vi "Process.vi"(8 "error in":errorcluster, 11 "Measurement.Free.UI":refnum<class "Measurement.Free.UI.lvclass">) -> (0 "error out":errorcluster, 3 "Measurement.Free.UI out":refnum<class "Measurement.Free.UI.lvclass">)   [LabVIEW 2017, in "Measurement.Free.UI.lvclass"]
doc: "---------------------------------------------------------------\nJKI State Machine Objects™\nhttp://jki.net/state-machine-objects/\nCopyright (C) 2005-2015, JKI <info@jki.net>\nALL RIGHTS RESERVEDJKI State Machine Objects (SMO) 1.0.0.5\nJKI - JKI\nCopyright (c) 2016, JKI"
uses:
  Measurement.Free.UI.lvclass
  D:/Program Files (x86)/National Instruments/LabVIEW 2017/vi.lib/JKI/JKI SMO/SMO/SMO.lvclass
  D:/Program Files (x86)/National Instruments/LabVIEW 2017/vi.lib/JKI/JKI SMO/SMO.UI/SMO.UI.lvclass
  <vilib>/JKI/JKI SMO/SMO/Typedefs/Parent Call--Enum.ctl
  Measurement.Free/Measurement.Free.lvclass
  D:/upwork/Laser Measurement Tool/Laser/project/Subsystems/Measurement/Measurement.lvclass
  Measurement.UI/Measurement.UI.lvclass
  <vilib>/JKI/JKI SMO/SMO/SMO.lvclass
  <vilib>/JKI/JKI SMO/SMO.UI/SMO.UI.lvclass
  Measurement/Measurement.lvclass
panel:
  in  "Set OPA Wavelength":bool
  in  "Set SMU Votage":bool
  in  "Shutter":bool
  in  "Wavelength, nm:":dbl=620.0
  in  "SMU Voltage, V:":dbl=1.0
  out "Initialized":bool
  out "Power monitor":cluster{"X":dbl, "Y":dbl}[](graph) caption="XY Graph - Dark"
  out "SMU":cluster{"X":dbl, "Y":dbl}[](graph) caption="XY Graph - Dark"
  out "LIA":cluster{"X":dbl, "Y":dbl}[](graph) caption="XY Graph - Dark"
  in  "Clear Button":bool
  in  "Pause Button":bool
  in  "Stop Button":bool
  in  "Start Button":bool
  in  "Close Button":bool
  # "SMU Control"
  # "OPA Control"
  # "For instructions on how to use the JKI State Machine Objects, examples and video tutorials, visit:\nhttp://jki.net/state-machine-objects/\n\nJKI State Machine Objects™\nhttp://jki.net/state-machine-objects/\nCopyright (C) 2005-2015, JKI <info@jki.net>\nALL RIGHTS RESERVED"
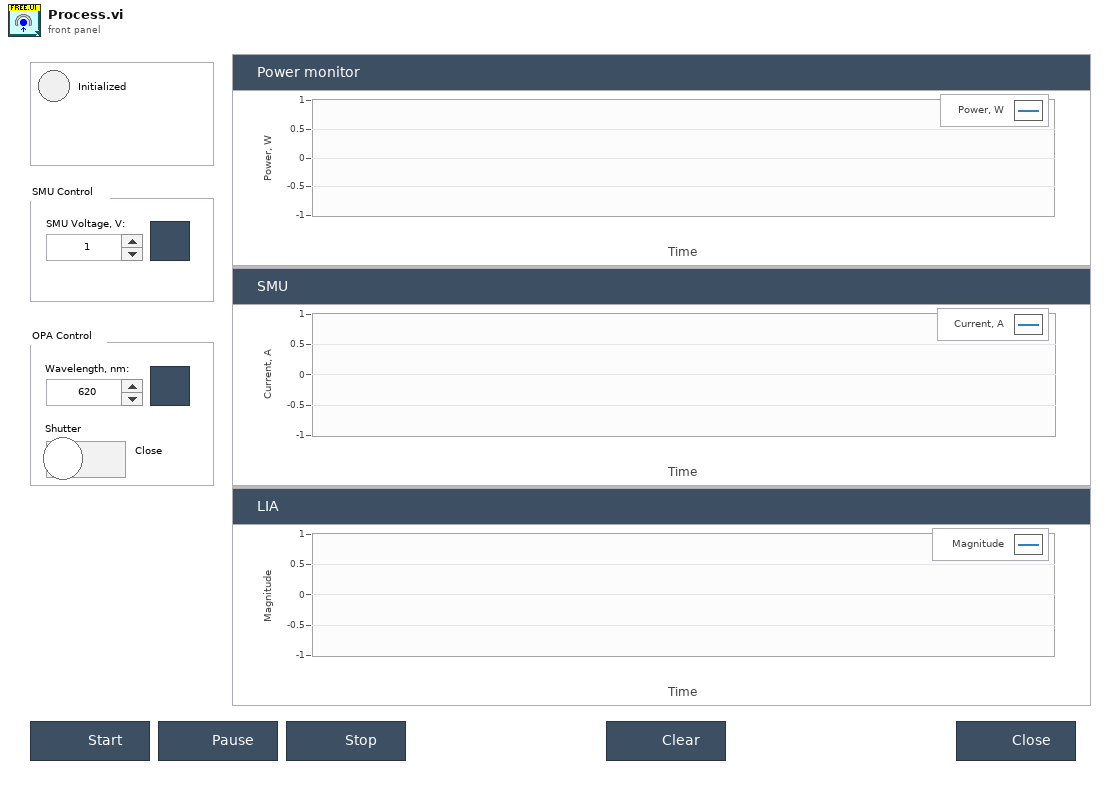
[diagram p1: front panel]
types:
  T1 = typedef "SMO.lvclass/Parent Call--Enum.ctl" = enum16{"Allows parent to run", "Does not request parent to run"}
  T2 = enum32{"invalid app kind", "Development System", "Run Time System", "Student Edition", "Embedded LabVIEW", "Evaluation", "Custom"}
  T3 = enum32{"Invalid", "Standard", "Closed", "Hidden", "Minimized", "Maximized"}
  T4 = typedef "Measurement.lvclass/PublicEvents--Measurement.Initialized.ctl" = bool
  T5 = enum8{"Enabled", "Disabled", "Disabled and Grayed Out"}
  T6 = typedef "Measurement.Free.UI.lvclass/Dependencies--Cluster.ctl" = cluster{"Measurement.Free":refnum<class "Measurement.Free.lvclass">}
  T7 = cluster{"Core":cluster{"Current VI Reference":refnum<vi>, "Close Panel on Exit?":bool, "error":errorcluster}, "Self Reference":refnum<class "Measurement.Free.UI.lvclass">, "Dependencies":T6, "SMU Data":cluster{"X":dbl, "Y":dbl}[], "LIA Data":cluster{"X":dbl, "Y":dbl}[], "OPM Data":cluster{"X":dbl, "Y":dbl}[]}
  T8 = cluster{"Current VI Reference":refnum<vi>, "Close Panel on Exit?":bool, "error":errorcluster}
  T9 = typedef "SMO.lvclass/Protected Events.ctl" = cluster{"StopProcesses":refnum<user-event>, "AbortProcesses":refnum<user-event>, "Config Changed":refnum<user-event>, "Dependency":refnum<user-event>}
  T10 = cluster{"Event Registration Refnum":refnum<event-registration>, "Measurement Public Events":refnum<event-registration>}
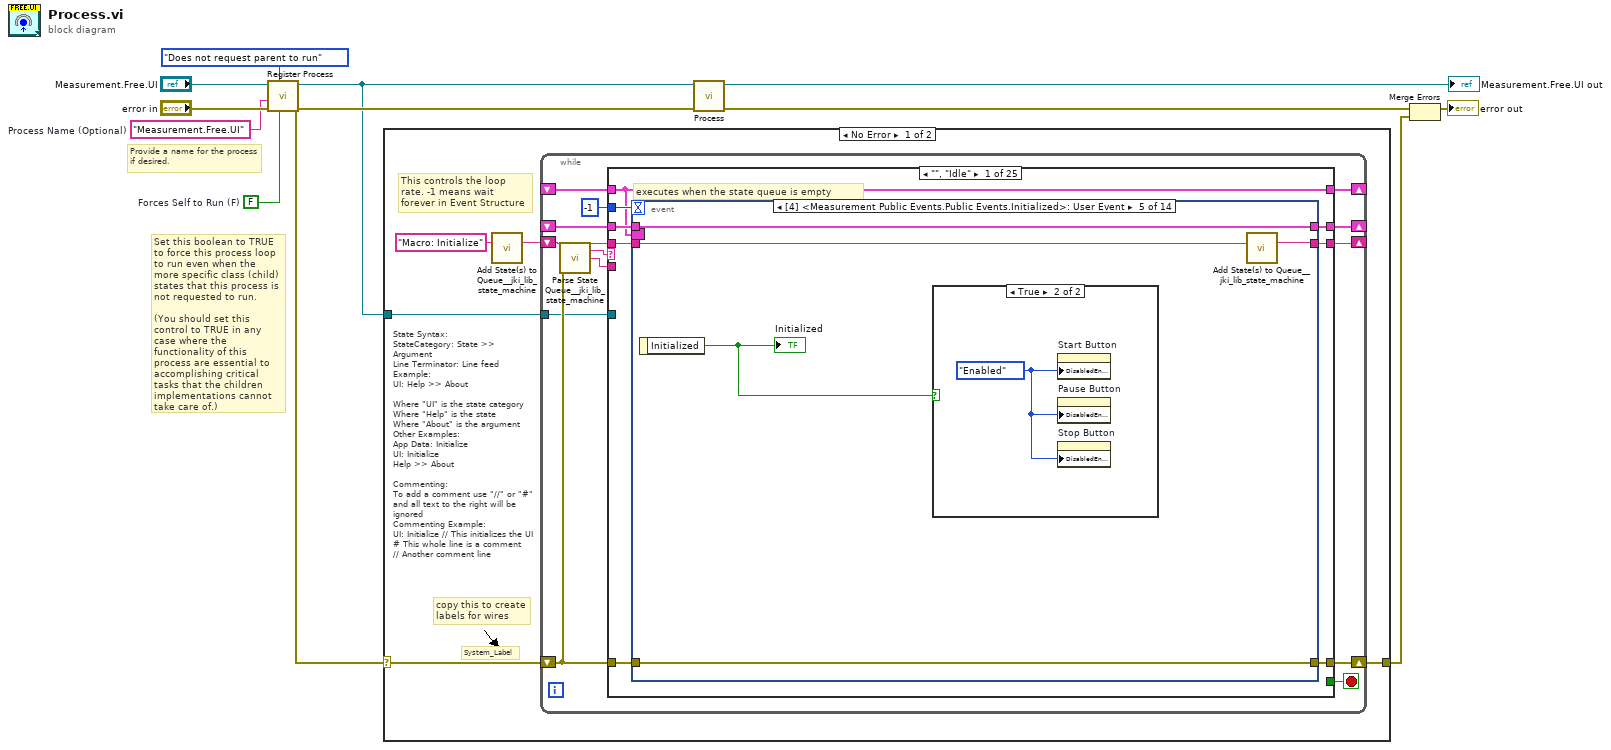
[diagram p0: block diagram]
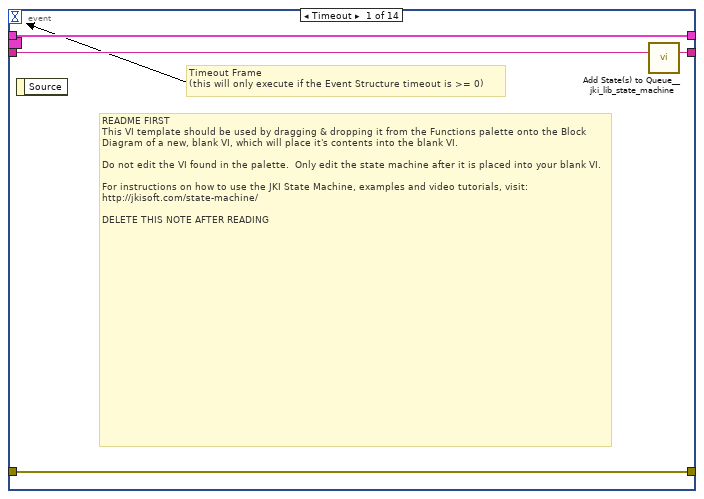
[diagram p2: hidden frame]
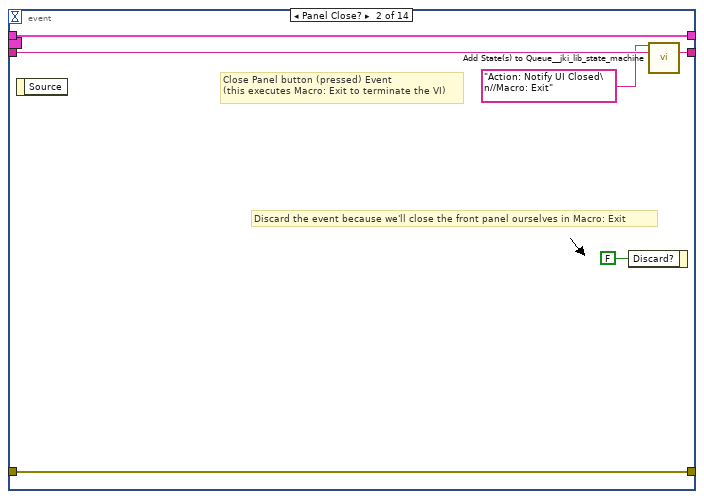
[diagram p3: hidden frame]
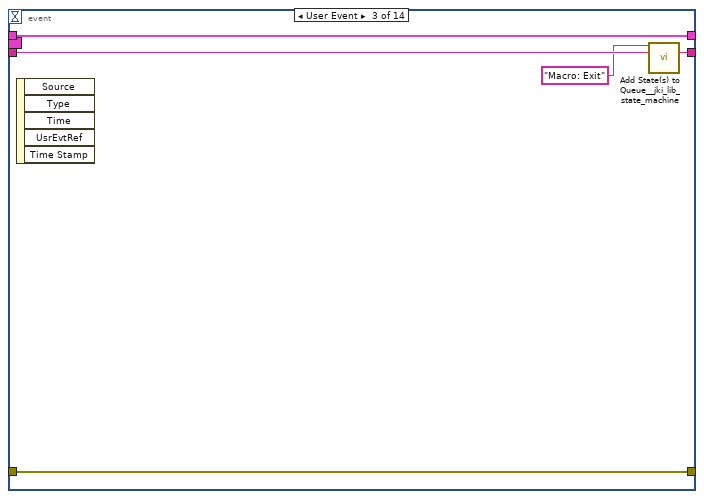
[diagram p4: hidden frame]
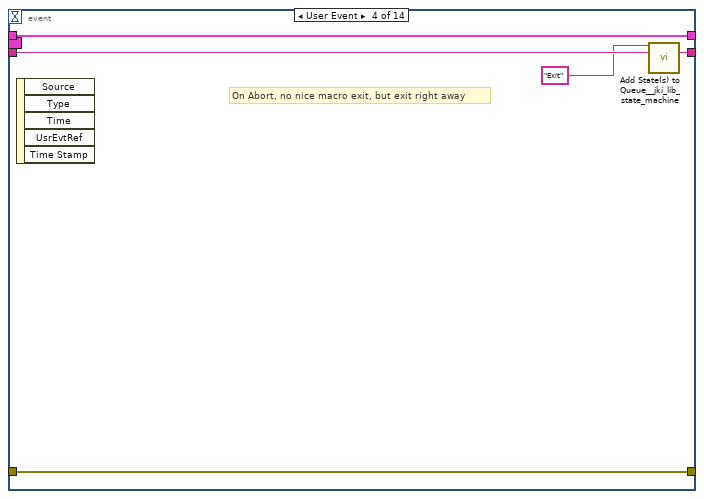
[diagram p5: hidden frame]
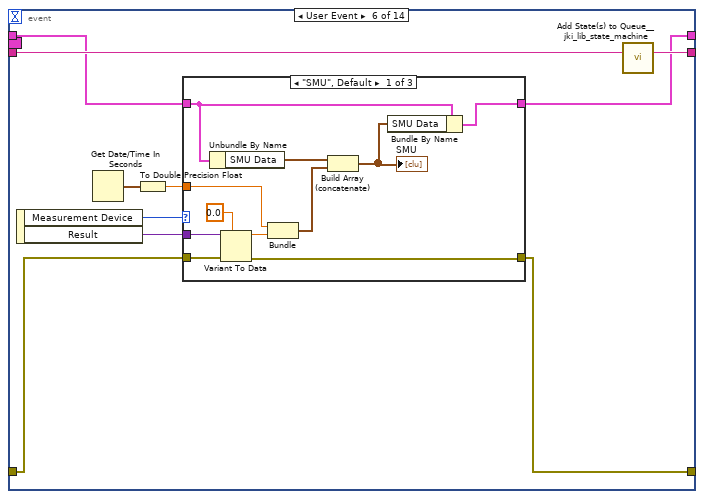
[diagram p7: hidden frame]
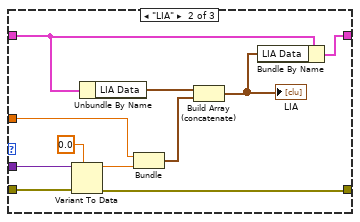
[diagram p8: hidden frame]
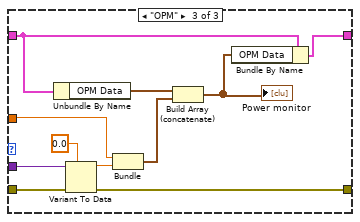
[diagram p9: hidden frame]
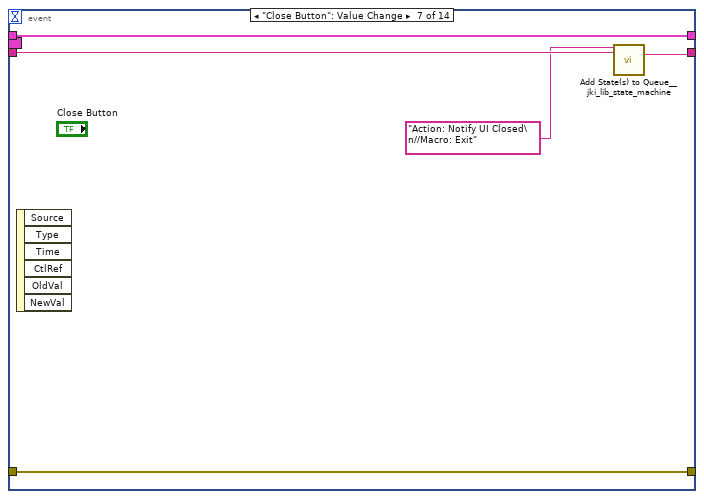
[diagram p10: hidden frame]
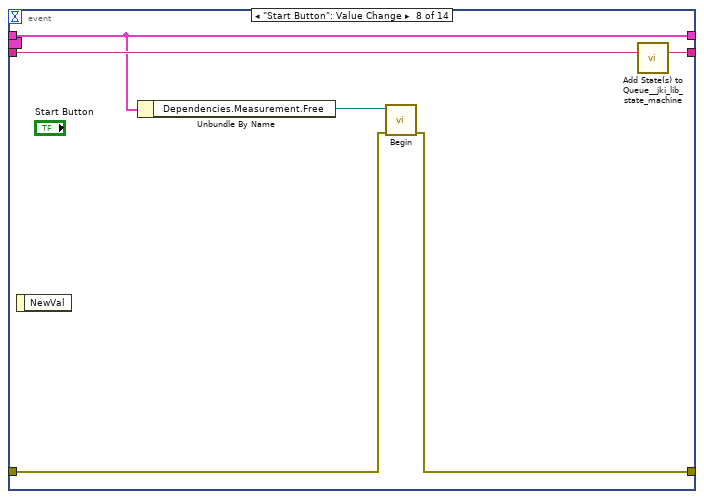
[diagram p11: hidden frame]
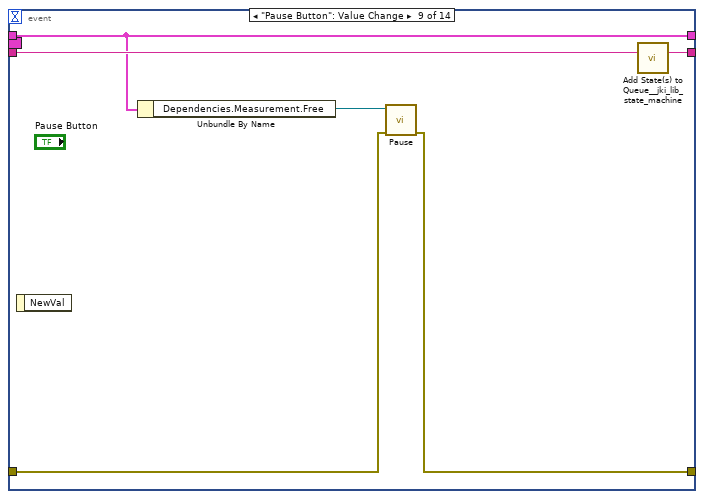
[diagram p12: hidden frame]
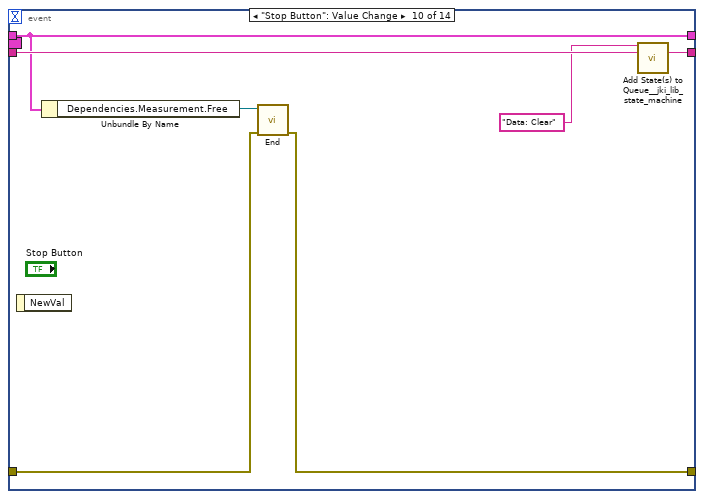
[diagram p13: hidden frame]
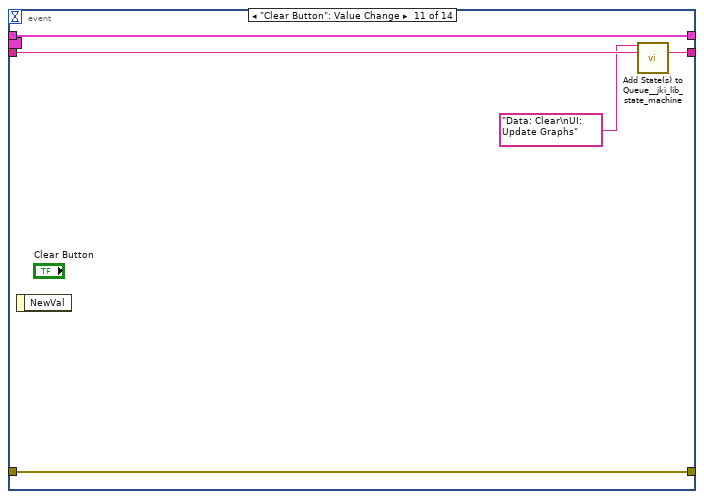
[diagram p14: hidden frame]
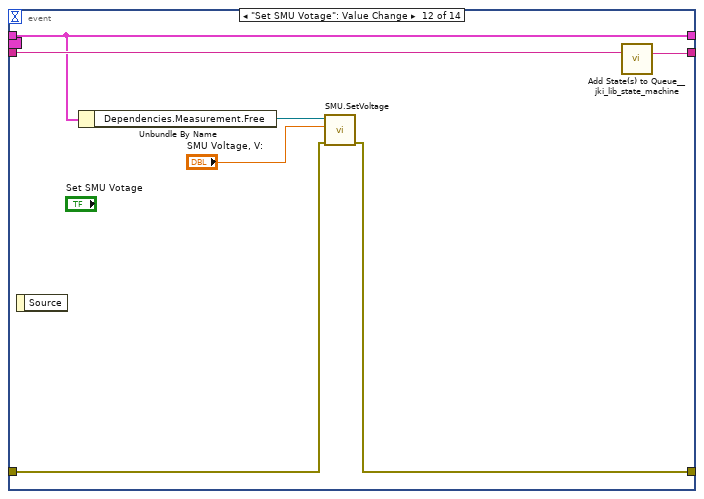
[diagram p15: hidden frame]
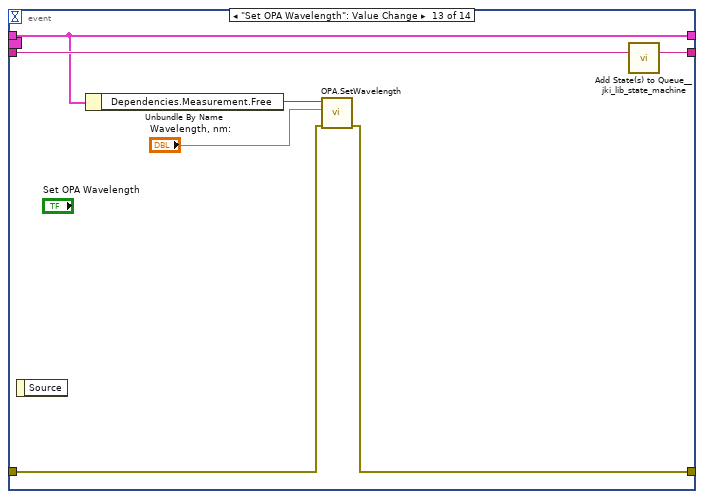
[diagram p16: hidden frame]
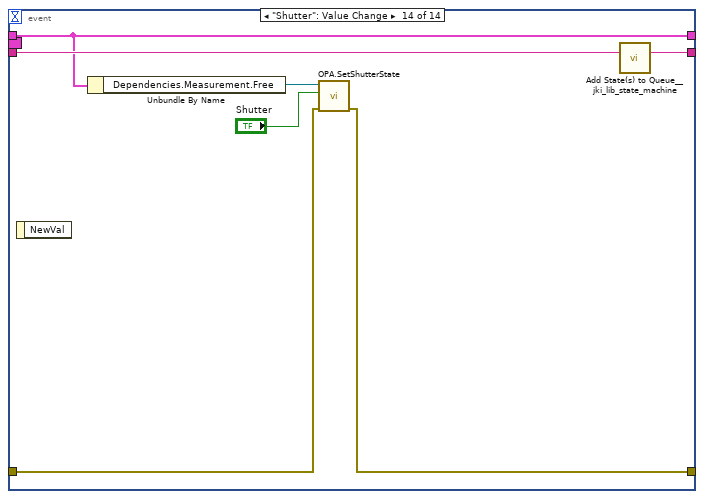
[diagram p17: hidden frame]
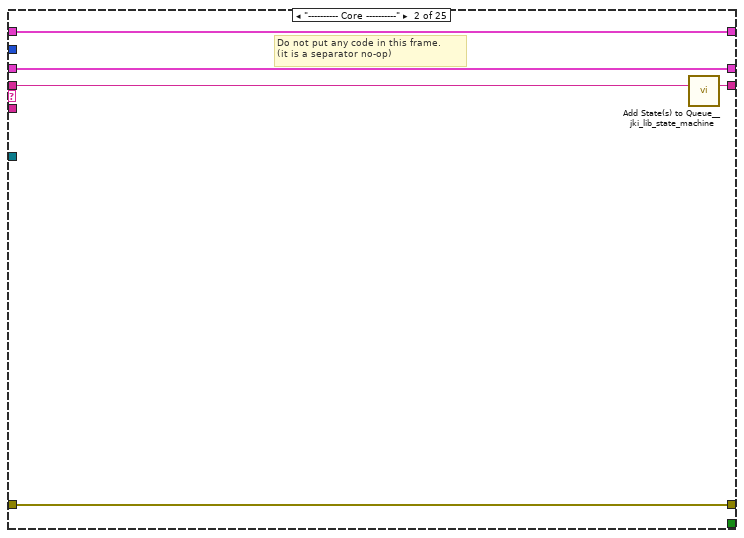
[diagram p18: hidden frame]
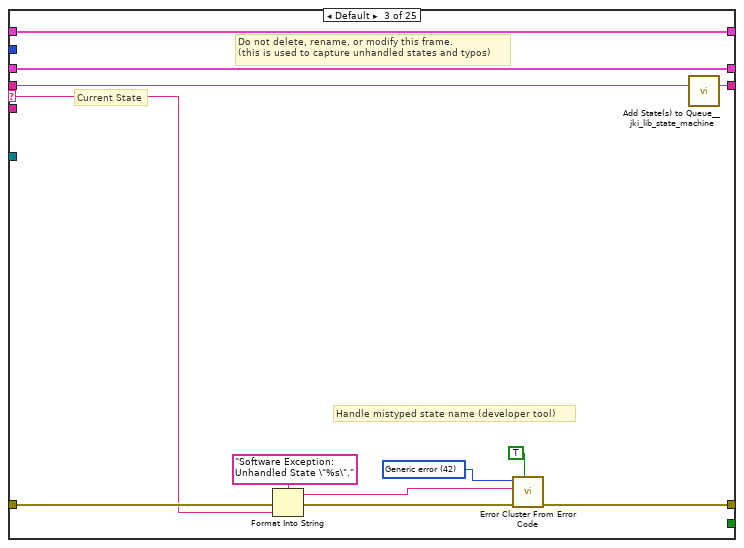
[diagram p19: hidden frame]
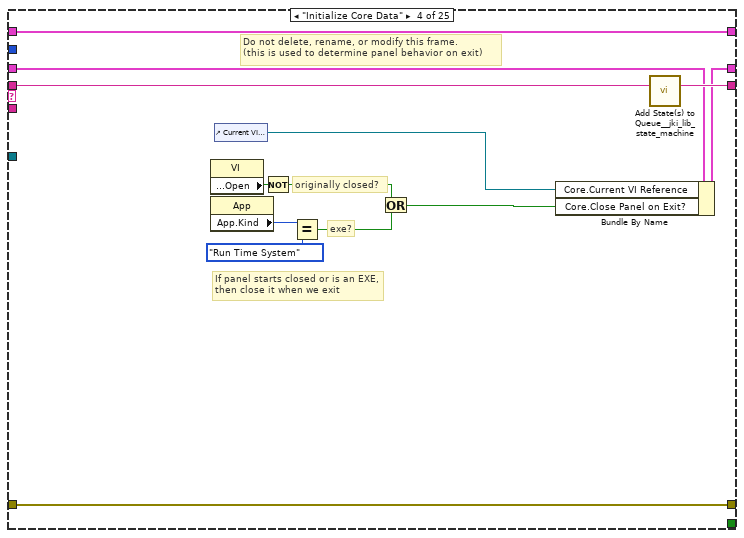
[diagram p20: hidden frame]
diagram:
  w2 = FALSE  # Forces Self to Run (F)
  w1 = "Measurement.Free.UI"  # Process Name (Optional)
  # "Provide a name for the process\nif desired."
  # "Set this boolean to TRUE to force this process loop to run even when the more specific class (child) states that this process is not requested to run.\n\n(You should set this control to TRUE in any case where the functionality of this process are essential to accomplishing critical tasks that the children implementations cannot take care of.)"
  n1 = call <vilib>:"Register Process.vi"("Forces Self to Run (F)"=w2, "Parent Call"=Parent_Call--Enum."Does not request parent to run", "error in (no error)"="error in", "Process Name (optional)"=w1, "SMO"="Measurement.Free.UI") -> ("error out"=w8:errorcluster, "SMO out"=w7:refnum<class "Measurement.Free.UI.lvclass">)  [unwired: 5 in]
  n2 = case shown="No Error" w8 {
    selector: w8 -> [w13 w402]
    tunnel: w7 -> [w14 _]
    tunnel: [w12 w402] -> w4
    frame No Error {
      # "State Syntax:\nStateCategory: State >> Argument\nLine Terminator: Line feed\nExample:\nUI: Help >> About\n\nWhere \"UI\" is the state category\nWhere \"Help\" is the state\nWhere \"About\" is the argument\nOther Examples:\nApp Data: Initialize\nUI: Initialize\nHelp >> About\n\nCommenting:\nTo add a comment use \"//\" or \"#\" and all text to the right will be ignored\nCommenting Example:\nUI: Initialize // This initializes the UI\n# This whole line is a comment\n// Another comment line"
      # "copy this to create labels for wires"
      # "This controls the loop rate. -1 means wait forever in Event Structure"
      # "System_Label"
      n3 = call <vilib>:"Add State(s) to Queue__jki_lib_state_machine.vi"("State(s) in (\"\")"="Macro: Initialize") -> ("States Out"=w16:string)  [unwired: 14 in]
      n4 = while {
        shift-right: [w23] -> _
        shift-left: _ -> [w22]
        shift-right: [w26] -> w12
        shift-left: w13 -> [w20]
        shift-right: [w25] -> _
        shift-left: w16 -> [w27]
        tunnel: w14 -> [w19]
        shift-right: [w18] -> _
        shift-left: _ -> [w17]
        stop <- w24 stop-if-true
        n5 = call <vilib>:"Parse State Queue__jki_lib_state_machine.vi"("State Queue"=w27, "Error In (no error)"=w20) -> ("Remaining States"=w29:string, "Current State"=w30:string, "Arguments"=w28:string)  [unwired: 11 in]
        n6 = case shown="\"\", \"Idle\"" w30 {
          selector: w30 -> [_ _ w164 _ _ _ _ _ _ _ _ _ _ _ _ _ _ _ _ _ _ _ _ _ _]
          tunnel: w29 -> [w38 w162 w168 w187 w201 w207 w212 w227 w234 w241 w246 w256 w263 w279 w318 w323 w332 w346 w351 w362 w367 w381 w387 w394 w401]
          tunnel: w28 -> [_ _ _ _ _ _ _ _ _ _ _ _ w257 w273 _ _ _ _ _ _ _ _ _ _ _]
          tunnel: w22 -> [w36 w159 w166 w178 w190 w203 w209 _ w230 w236 w243 w254 w261 w275 w315 w320 w328 w337 w348 w359 w364 w373 w385 w390 w397]
          tunnel: [w35 w160 w170 w184 w192 w202 w210 w217 w232 w237 w244 w250 w258 w276 w307 w321 w330 w344 w349 w353 w365 w376 w382 w391 w395] -> w26
          tunnel: w20 -> [w34 w160 w169 w184 w197 _ w210 w224 w232 w238 w244 w248 w259 w277 w311 w321 w330 w344 w349 w354 w365 w378 w383 w391 w396]
          tunnel: [w37 w161 w167 w186 w200 w206 w211 w226 w233 w240 w245 w255 w262 w278 w317 w322 w331 w345 w350 w361 w366 w380 w386 w393 w400] -> w25
          tunnel: [_ _ _ _ _ TRUE _ _ _ _ _ _ _ _ _ _ _ _ _ _ _ _ _ _ _] -> w24
          tunnel: [w33 w159 w166 w185 w189 w203 w209 w225 w228 w236 w243 w254 w261 w275 w315 w320 w328 w337 w348 w359 w364 w373 w385 w389 w397] -> w23
          tunnel: -1 ("Timeout") -> [w32 _ _ _ _ _ _ _ _ _ _ _ _ _ _ _ _ _ _ _ _ _ _ _ _]
          tunnel: w19 -> [_ _ _ _ _ _ _ w222 _ _ _ _ _ _ _ _ _ _ _ _ _ _ _ _ _]
          tunnel: [w31 w158 w163 w175 w199 w204 w208 w221 w231 w235 w242 w253 w260 w272 w316 w319 w329 w338 w347 w360 w363 w371 w384 w392 w399] -> w18
          tunnel: w17 -> [w31 w158 w163 w175 w199 w204 w208 w221 w231 w235 w242 w253 w260 w272 w316 w319 w329 w338 w347 w360 w363 _ w384 w392 w399]
          frame "", "Idle" {
            # "executes when the state queue is empty"
            n7 = event shown="[4] <Measurement Public Events.Public Events.Initialized>: User Event" {
              selector: w31 -> [_ _ _ _ _ _ _ _ _ _ _ _ _ _]
              dyn-events: _ -> [_ _ _ _ _ _ _ _ _ _ _ _ _ _]
              timeout: w32 -> [_ _ _ _ _ _ _ _ _ _ _ _ _ _]
              tunnel: w38 -> [w42 w48 w53 w58 w61 w73 w110 w118 w124 w131 w136 w142 w149 w156]
              tunnel: [w41 w47 w52 w57 w62 w74 w111 w117 w123 w130 w135 w143 w150 w157] -> w37
              tunnel: w36 -> [w39 w44 w50 w55 w63 w70 w109 w116 w122 w129 w134 w141 w148 w155]
              tunnel: [w40 w43 w51 w56 w60 w65 w112 w113 w119 w126 w132 w137 w144 w151] -> w35
              tunnel: w34 -> [w40 w43 w51 w56 w60 w66 w112 w114 w120 w127 w132 w138 w145 w152]
              tunnel: [w39 w44 w50 w55 w63 w69 w109 w116 w122 w129 w134 w141 w148 w155] -> w33
              event Timeout {
                # "README FIRST\nThis VI template should be used by dragging & dropping it from the Functions palette onto the Block Diagram of a new, blank VI, which will place it's contents into the blank VI.\n\nDo not edit the VI found in the palette.  Only edit the state machine after it is placed into your blank VI.\n\nFor instructions on how to use the JKI State Machine, examples and video tutorials, visit:\nhttp://jkisoft.com/state-machine/\n\nDELETE THIS NOTE AFTER READING"
                # "Timeout Frame\n(this will only execute if the Event Structure timeout is >= 0)"
                n8 = event-data() -> ()  [unwired: 1 in, 1 out]
                n9 = call <vilib>:"Add State(s) to Queue__jki_lib_state_machine.vi"("State(s) in (\"\")"=w42) -> ("States Out"=w41:string)  [unwired: 14 in]
              }
              event Panel Close? {
                # "Discard the event because we'll close the front panel ourselves in Macro: Exit"
                # "Close Panel button (pressed) Event\n(this executes Macro: Exit to terminate the VI)"
                n10 = event-data() -> ()  [unwired: 1 in, 1 out]
                n11 = event-data("Discard?"=FALSE) -> ()  [unwired: 1 in, 1 out]
                n12 = call <vilib>:"Add State(s) to Queue__jki_lib_state_machine.vi"("State(s) in Front (\"\")"="Action: Notify UI Closed\n//Macro: Exit", "State(s) in (\"\")"=w48) -> ("States Out"=w47:string)  [unwired: 13 in]
              }
              event User Event {
                n13 = event-data() -> ()  [unwired: 1 in, 5 out]
                n14 = call <vilib>:"Add State(s) to Queue__jki_lib_state_machine.vi"("State(s) in Front (\"\")"="Macro: Exit", "State(s) in (\"\")"=w53) -> ("States Out"=w52:string)  [unwired: 13 in]
              }
              event User Event {
                # "On Abort, no nice macro exit, but exit right away"
                n15 = event-data() -> ()  [unwired: 1 in, 5 out]
                n16 = call <vilib>:"Add State(s) to Queue__jki_lib_state_machine.vi"("State(s) in Front (\"\")"="Exit", "State(s) in (\"\")"=w58) -> ("States Out"=w57:string)  [unwired: 13 in]
              }
              event User Event {
                n17 = event-data() -> ("Initialized"=w59:T4)  [unwired: 1 in]
                "Initialized" <- w59
                n18 = case shown="True" w59 {
                  frame False {
                  }
                  frame True {
                    w64 = T5."Enabled" ("Disabled")
                    n19 = property on="Start Button" class="Bool"("DisabledEnum"=w64) -> ()  [unwired: 2 in, 2 out]
                    n20 = property on="Pause Button" class="Bool"("DisabledEnum"=w64) -> ()  [unwired: 2 in, 2 out]
                    n21 = property on="Stop Button" class="Bool"("DisabledEnum"=w64) -> ()  [unwired: 2 in, 2 out]
                  }
                }
                n22 = call <vilib>:"Add State(s) to Queue__jki_lib_state_machine.vi"("State(s) in (\"\")"=w61) -> ("States Out"=w62:string)  [unwired: 14 in]
              }
              event User Event {
                n23 = event-data() -> ("Measurement Device"=w72:enum16{"SMU", "LIA", "OPM"}, "Result"=w71:variant)  [unwired: 1 in]
                n24 = Get Date/Time In Seconds() -> (seconds since 1Jan1904=w68:timestamp)
                n25 = To Double Precision Float(number=w68) -> (double precision float=w67:dbl)
                n26 = case shown="\"SMU\", Default" w72 {
                  tunnel: w71 -> [w84 w95 w106]
                  tunnel: w70 -> [w80 w90 w103]
                  tunnel: [w77 w89 w102] -> w69
                  tunnel: w67 -> [w78 w92 w100]
                  tunnel: w66 -> [w76 w87 w98]
                  tunnel: [w75 w86 w97] -> w65
                  frame "SMU", Default {
                    n27 = Unbundle By Name(w80) -> ("SMU Data"=w81:cluster{"X":dbl, "Y":dbl}[])
                    n28 = Variant To Data(error in=w76, type=0.0, Variant=w84) -> (data=w83:dbl, error out=w75:errorcluster)
                    n29 = Bundle(w78, w83) -> (w82:cluster{dbl, dbl})  [unwired: 1 in]
                    n30 = Build Array (concatenate)(w81, w82) -> (w79:cluster{"X":dbl, "Y":dbl}[])
                    "SMU" <- w79
                    n31 = Bundle By Name(cluster=w80, "SMU Data"=w79) -> (w77:T7)
                  }
                  frame "LIA" {
                    n32 = Variant To Data(error in=w87, type=0.0, Variant=w95) -> (data=w91:dbl, error out=w86:errorcluster)
                    n33 = Unbundle By Name(w90) -> ("LIA Data"=w93:cluster{"X":dbl, "Y":dbl}[])
                    n34 = Bundle(w92, w91) -> (w94:cluster{dbl, dbl})  [unwired: 1 in]
                    n35 = Build Array (concatenate)(w93, w94) -> (w88:cluster{"X":dbl, "Y":dbl}[])
                    "LIA" <- w88
                    n36 = Bundle By Name(cluster=w90, "LIA Data"=w88) -> (w89:T7)
                  }
                  frame "OPM" {
                    n37 = Unbundle By Name(w103) -> ("OPM Data"=w104:cluster{"X":dbl, "Y":dbl}[])
                    n38 = Variant To Data(error in=w98, type=0.0, Variant=w106) -> (data=w99:dbl, error out=w97:errorcluster)
                    n39 = Bundle(w100, w99) -> (w105:cluster{dbl, dbl})  [unwired: 1 in]
                    n40 = Build Array (concatenate)(w104, w105) -> (w101:cluster{"X":dbl, "Y":dbl}[])
                    "Power monitor" <- w101
                    n41 = Bundle By Name(cluster=w103, "OPM Data"=w101) -> (w102:T7)
                  }
                }
                n42 = call <vilib>:"Add State(s) to Queue__jki_lib_state_machine.vi"("State(s) in (\"\")"=w73) -> ("States Out"=w74:string)  [unwired: 14 in]
              }
              event "Close Button": Value Change {
                n43 = event-data() -> ()  [unwired: 1 in, 6 out]
                n44 = call <vilib>:"Add State(s) to Queue__jki_lib_state_machine.vi"("State(s) in Front (\"\")"="Action: Notify UI Closed\n//Macro: Exit", "State(s) in (\"\")"=w110) -> ("States Out"=w111:string)  [unwired: 13 in]
              }
              event "Start Button": Value Change {
                n45 = event-data() -> ()  [unwired: 1 in, 1 out]
                n46 = Unbundle By Name(w116) -> ("Dependencies.Measurement.Free"=w115:refnum<class "Measurement.Free.lvclass">)
                n47 = call "Begin.vi"("error in (no error)"=w114, "Measurement in"=w115) -> ("error out"=w113:errorcluster)  [unwired: 8 in, 1 out]
                n48 = call <vilib>:"Add State(s) to Queue__jki_lib_state_machine.vi"("State(s) in (\"\")"=w118) -> ("States Out"=w117:string)  [unwired: 14 in]
              }
              event "Pause Button": Value Change {
                n49 = event-data() -> ()  [unwired: 1 in, 1 out]
                n50 = Unbundle By Name(w122) -> ("Dependencies.Measurement.Free"=w121:refnum<class "Measurement.Free.lvclass">)
                n51 = call "Pause.vi"("error in (no error)"=w120, "Measurement in"=w121) -> ("error out"=w119:errorcluster)  [unwired: 8 in, 1 out]
                n52 = call <vilib>:"Add State(s) to Queue__jki_lib_state_machine.vi"("State(s) in (\"\")"=w124) -> ("States Out"=w123:string)  [unwired: 14 in]
              }
              event "Stop Button": Value Change {
                n53 = event-data() -> ()  [unwired: 1 in, 1 out]
                n54 = Unbundle By Name(w129) -> ("Dependencies.Measurement.Free"=w128:refnum<class "Measurement.Free.lvclass">)
                n55 = call "End.vi"("error in (no error)"=w127, "Measurement in"=w128) -> ("error out"=w126:errorcluster)  [unwired: 8 in, 1 out]
                n56 = call <vilib>:"Add State(s) to Queue__jki_lib_state_machine.vi"("State(s) in Front (\"\")"="Data: Clear", "State(s) in (\"\")"=w131) -> ("States Out"=w130:string)  [unwired: 13 in]
              }
              event "Clear Button": Value Change {
                n57 = event-data() -> ()  [unwired: 1 in, 1 out]
                n58 = call <vilib>:"Add State(s) to Queue__jki_lib_state_machine.vi"("State(s) in Front (\"\")"="Data: Clear\nUI: Update Graphs", "State(s) in (\"\")"=w136) -> ("States Out"=w135:string)  [unwired: 13 in]
              }
              event "Set SMU Votage": Value Change {
                n59 = event-data() -> ()  [unwired: 1 in, 1 out]
                n60 = Unbundle By Name(w141) -> ("Dependencies.Measurement.Free"=w140:refnum<class "Measurement.Free.lvclass">)
                n61 = call "SMU.SetVoltage.vi"("error in (no error)"=w138, "Voltage, V"="SMU Voltage, V:", "Measurement.Free"=w140) -> ("error out"=w137:errorcluster)  [unwired: 7 in, 1 out]
                n62 = call <vilib>:"Add State(s) to Queue__jki_lib_state_machine.vi"("State(s) in (\"\")"=w142) -> ("States Out"=w143:string)  [unwired: 14 in]
              }
              event "Set OPA Wavelength": Value Change {
                n63 = event-data() -> ()  [unwired: 1 in, 1 out]
                n64 = Unbundle By Name(w148) -> ("Dependencies.Measurement.Free"=w147:refnum<class "Measurement.Free.lvclass">)
                n65 = call "OPA.SetWavelength.vi"("error in (no error)"=w145, "Wavelength, nm"="Wavelength, nm:", "Measurement.Free"=w147) -> ("error out"=w144:errorcluster)  [unwired: 7 in, 1 out]
                n66 = call <vilib>:"Add State(s) to Queue__jki_lib_state_machine.vi"("State(s) in (\"\")"=w149) -> ("States Out"=w150:string)  [unwired: 14 in]
              }
              event "Shutter": Value Change {
                n67 = event-data() -> ()  [unwired: 1 in, 1 out]
                n68 = Unbundle By Name(w155) -> ("Dependencies.Measurement.Free"=w154:refnum<class "Measurement.Free.lvclass">)
                n69 = call "OPA.SetShutterState.vi"("error in (no error)"=w152, "Shutter State"="Shutter", "Measurement.Free"=w154) -> ("error out"=w151:errorcluster)  [unwired: 7 in, 1 out]
                n70 = call <vilib>:"Add State(s) to Queue__jki_lib_state_machine.vi"("State(s) in (\"\")"=w156) -> ("States Out"=w157:string)  [unwired: 14 in]
              }
            }
          }
          frame "---------- Core ----------" {
            # "Do not put any code in this frame.\n(it is a separator no-op)"
            n71 = call <vilib>:"Add State(s) to Queue__jki_lib_state_machine.vi"("State(s) in (\"\")"=w162) -> ("States Out"=w161:string)  [unwired: 14 in]
          }
          frame Default {
            w173 = 42 items=["No error", "Argument error", "Memory is full", "Out of zone", "End of file", "File already open", "Generic file I/O error", "File not found", "File permission error", "Disk is full", "Duplicate path", "Too many files open", "System feature not enabled", "Resource file not found", "Cannot add resource", "Resource not found", "Image not found", "Image memory error", "Pen does not exist", "Config type invalid", "Config token not found", "Config parse error", "Config memory error", "Bad external code format", "Bad external code offset", "External code not present", "Null window", "Destroy window error", "Null menu", "Print aborted", "Bad print record", "Print driver error", "Windows error during printing", "Memory error during printing", "Print dialog error", "Generic print error", "Invalid device refnum", "Device not found", "Device parameter error", "Device unit error", "Cannot open device", "Device call aborted", "Generic error", "Cancelled by user", "Object ID too low", "Object ID too high", "Object not in heap", "Unknown heap", "Unknown object (invalid DefProc)", "Unknown object (DefProc not in table)", "Message out of range", "Invalid (null) method", "Unknown message", "Manager call not supported", "Bad address", "Network operation in progress", "Network operation timed out", "Connection is busy", "Network attribute not supported", "Network error", "Address in use", "System out of memory", "Connection aborted", "Connection refused", "Not connected", "Already connected", "Connection closed", "Initialization error (interapplication manager)", "Bad occurrence", "Wait on unbound occurrence handler", "Occurrence queue overflow", "Datalog type conflict", "Unused", "Unrecognized type (interapplication manager)", "Memory corrupt", "Failed to make temporary DLL", "Old CIN version", "Drag socket not found", "Failed to load drop-object", "Failed to register OLE object", "Failed to release OLE object", "Format specifier type mismatch", "Unknown format specifier", "Too few format specifiers", "Too many format specifiers", "Scan failed", "Newer CIN version", "Error converting to variant", "Runtime menu error", "Password tampered", "Variant attribute not found", "Incompatible variant data type", "Event data is not available", "Event Store is not present", "Occurrence is not found", "Event Queue is not created", "Event info is not available", "Refnum passed is NULL", "Error retrieving Class GUID", "Error retrieving CoClass GUID", "Error retrieving TypeLib GUID.", "Bad built application magic bytes.", "Specific driver is different from the specific driver associated with the Logical Name.", "There is no session opened to the class driver.", "Max Error", "MAX - Error with config objects", "MAX - Error loading configuration", "MAX - Group not supported"]
            # "Current State"
            # "Do not delete, rename, or modify this frame.\n(this is used to capture unhandled states and typos)"
            # "Handle mistyped state name (developer tool)"
            n72 = Format Into String(format string="Software Exception: Unhandled State \"%s\"." ("message"), error in=w169, w164) -> (resulting string=w172:string, error out=w171:errorcluster)  [unwired: 1 in]
            n73 = call <vilib>:"Error Cluster From Error Code.vi"("show call chain? (False)"=TRUE, "error in (no error)"=w171, "error message (\"\")"=w172, "error code (0)"=w173) -> ("error out"=w170:errorcluster)  [unwired: 5 in]
            n74 = call <vilib>:"Add State(s) to Queue__jki_lib_state_machine.vi"("State(s) in (\"\")"=w168) -> ("States Out"=w167:string)  [unwired: 14 in]
          }
          frame "Initialize Core Data" {
            # "Do not delete, rename, or modify this frame.\n(this is used to determine panel behavior on exit)"
            # "originally closed?"
            # "exe?"
            # "If panel starts closed or is an EXE, then close it when we exit"
            n75 = property class="VI"() -> ("Front Panel.Open"=w183:bool)  [unwired: 2 in, 2 out]
            n76 = property class="App"() -> ("App.Kind"=w182:T2)  [unwired: 2 in, 2 out]
            n77 = control-ref of="Current VI Reference"() -> (w176:refnum<vi>)
            n78 = Not(x=w183) -> (.not. x?=w180:bool)
            n79 = Equal?(x=w182, y=T2."Run Time System" ("Application:Kind")) -> (x = y?=w179:bool)
            n80 = Or(x=w180, y=w179) -> (x .or. y?=w177:bool)
            n81 = Bundle By Name(cluster=w178, "Core.Current VI Reference"=w176, "Core.Close Panel on Exit?"=w177) -> (w185:T7)
            n82 = call <vilib>:"Add State(s) to Queue__jki_lib_state_machine.vi"("State(s) in (\"\")"=w187) -> ("States Out"=w186:string)  [unwired: 14 in]
          }
          frame "Error Handler" {
            w192 = errorcluster {"status"=FALSE, "code"=0, "source"=""}  # No error
            # "Overwrite this method to handle errors and pass to parent if not handled. Parent will fire a public event if the error is not handled up the chain of classes."
            # "Handle any errors here.\nYou can also output any states to clean-up after errors occur"
            n83 = Unbundle By Name(w190) -> ("Self Reference"=w198:refnum<class "Measurement.Free.UI.lvclass">)
            n84 = call-dynamic "Handle Error.vi"("Stop on Unhandled Error (T)"=TRUE, "error in"=w197, "SMO"=w198) -> ("handling error"=w193:errorcluster, "Unhandled error"=w191:errorcluster)  [unwired: 6 in, 1 out]
            n85 = Bundle By Name(cluster=w190, "Core.error"=w191) -> (w189:T7)
            n86 = Select(t="Exit", s=w193, f="") -> (s? t:f=w194:string)
            n87 = call <vilib>:"Add State(s) to Queue__jki_lib_state_machine.vi"("State(s) in Front (\"\")"=w194, "State(s) in (\"\")"=w201) -> ("States Out"=w200:string)  [unwired: 13 in]
          }
          frame "Exit" {
            # "Do not put any code in this frame.\n(No errors that occur here will be handled.)"
            n88 = Unbundle By Name(w203) -> ("Core.error"=w202:errorcluster)
            n89 = call <vilib>:"Add State(s) to Queue__jki_lib_state_machine.vi"("State(s) in (\"\")"=w207) -> ("States Out"=w206:string)  [unwired: 14 in]
          }
          frame "---------- Data ----------" {
            # "Do not put any code in this frame.\n(It is a separator no-op. You can make a copy of this frame to create a new Data frame)"
            n90 = call <vilib>:"Add State(s) to Queue__jki_lib_state_machine.vi"("State(s) in (\"\")"=w212) -> ("States Out"=w211:string)  [unwired: 14 in]
          }
          frame "Data: Initialize" {
            w213 = cluster{"X":dbl, "Y":dbl}[] []  # OPM Data
            w214 = cluster{"X":dbl, "Y":dbl}[] []  # LIA Data
            w215 = cluster{"X":dbl, "Y":dbl}[] []  # SMU Data
            w220 = T8 {"Current VI Reference"=refnum, "Close Panel on Exit?"=FALSE, "error"={"status"=FALSE, "code"=0, "source"=""}}  # Core
            w223 = refnum<class "Measurement.Free.UI.lvclass"> refnum  # Self Reference
            # "do not delete - used by framework"
            # "Expand Bundle to add new data elements to shift register data."
            # "Data names and types of shift register data are defined by this bundle."
            # "Initialize the shift-register data, here.\n(data names are defined by what you wire into the bundle function)"
            n91 = Variant To Data(error in=w224, type=w223, Variant=w222) -> (data=w219:refnum<class "Measurement.Free.UI.lvclass">, error out=w218:errorcluster)
            n92 = call "Measurement.Free.UI.GetDependencies.vi"("error in (no error)"=w218, "Measurement.Free.UI in"=w219) -> ("error out"=w217:errorcluster, "Dependencies"=w216:T6)  [unwired: 7 in, 1 out]
            n93 = Bundle("Core"=w220, "Self Reference"=w219, "Dependencies"=w216, "SMU Data"=w215, "LIA Data"=w214, "OPM Data"=w213) -> (w225:T7)  [unwired: 1 in]
            n94 = call <vilib>:"Add State(s) to Queue__jki_lib_state_machine.vi"("State(s) in (\"\")"=w227) -> ("States Out"=w226:string)  [unwired: 14 in]
          }
          frame "Data: Clear" {
            w229 = cluster{"X":dbl, "Y":dbl}[] [] ("SMU Data")
            n95 = Bundle By Name(cluster=w230, "SMU Data"=w229, "LIA Data"=w229, "OPM Data"=w229) -> (w228:T7)
            n96 = call <vilib>:"Add State(s) to Queue__jki_lib_state_machine.vi"("State(s) in (\"\")"=w234) -> ("States Out"=w233:string)  [unwired: 14 in]
          }
          frame "Data: Cleanup" {
            # "Cleanup any data and references, here.\n(this is called automatically, by the Macro: Exit)"
            n97 = Unbundle By Name(w236) -> ("Core.Current VI Reference"=w239:refnum<vi>)
            n98 = Close Reference(reference=w239, error in (no error)=w238) -> (error out=w237:errorcluster)
            n99 = call <vilib>:"Add State(s) to Queue__jki_lib_state_machine.vi"("State(s) in (\"\")"=w241) -> ("States Out"=w240:string)  [unwired: 14 in]
          }
          frame "---------- UI ----------" {
            # "Do not put any code in this frame.\n(It is a separator no-op. You can make a copy of this frame to create a new UI frame)"
            n100 = call <vilib>:"Add State(s) to Queue__jki_lib_state_machine.vi"("State(s) in (\"\")"=w246) -> ("States Out"=w245:string)  [unwired: 14 in]
          }
          frame "UI: Initialize" {
            w247 = T5."Disabled and Grayed Out" ("Disabled")
            # "Initialize the User Interface, here.\n(this is called automatically, by the Macro: Init)"
            n101 = invoke on="Initialized" class="Bool (strict)" method="Reinit To Default"(error in=w248) -> (error out=w249:errorcluster)  [unwired: 2 in, 2 out]
            n102 = invoke on="Power monitor" class="XYGraph (strict)" method="Reinit To Default"(error in=w249) -> (error out=w252:errorcluster)  [unwired: 2 in, 2 out]
            n103 = invoke on="SMU" class="XYGraph (strict)" method="Reinit To Default"(error in=w252) -> (error out=w251:errorcluster)  [unwired: 2 in, 2 out]
            n104 = property on="Start Button" class="Bool"("DisabledEnum"=w247) -> ()  [unwired: 2 in, 2 out]
            n105 = property on="Pause Button" class="Bool"("DisabledEnum"=w247) -> ()  [unwired: 2 in, 2 out]
            n106 = property on="Stop Button" class="Bool"("DisabledEnum"=w247) -> ()  [unwired: 2 in, 2 out]
            n107 = invoke on="LIA" class="XYGraph (strict)" method="Reinit To Default"(error in=w251) -> (error out=w250:errorcluster)  [unwired: 2 in, 2 out]
            n108 = call <vilib>:"Add State(s) to Queue__jki_lib_state_machine.vi"("State(s) in (\"\")"=w256) -> ("States Out"=w255:string)  [unwired: 14 in]
          }
          frame "UI: Cursor Set" {
            # "Argument"
            # "Initialize the User Interface, here.\n(this is called automatically, by the Macro: Init)"
            n109 = disable-structure shown="Default" {
              disable-tunnel: w259 -> [w264 w267]
              disable-tunnel: [w264 w266] -> w258
              disable-tunnel: w257 -> [_ w265]
              frame condition #0 {
              }
              frame condition #1 (active) {
                n110 = case shown="\"Idle\", Default" w265 {
                  tunnel: w267 -> [w269 w271]
                  tunnel: [w268 w270] -> w266
                  frame "Idle", Default {
                    n111 = call <vilib>:"Unset Busy.vi"("error in (no error)"=w269) -> ("error out"=w268:errorcluster)  [unwired: 10 in]
                  }
                  frame "Busy" {
                    n112 = call <vilib>:"Set Busy.vi"("error in (no error)"=w271) -> ("error out"=w270:errorcluster)  [unwired: 9 in, 1 out]
                  }
                }
              }
            }
            n113 = call <vilib>:"Add State(s) to Queue__jki_lib_state_machine.vi"("State(s) in (\"\")"=w263) -> ("States Out"=w262:string)  [unwired: 14 in]
          }
          frame "UI: Front Panel State" {
            # "Argument"
            # "Set Front Panel Open or Closed\n(Usage: \"UI: Front Panel State >> Open|Close\")"
            n114 = Unbundle By Name(w275) -> ("Core.Current VI Reference"=w274:refnum<vi>)
            n115 = disable-structure shown="Default" {
              disable-tunnel: w277 -> [w283 w306]
              disable-tunnel: [w282 w306] -> w276
              disable-tunnel: w274 -> [w281 _]
              disable-tunnel: w273 -> [w280 _]
              frame condition #0 (active) {
                n116 = case shown="\"Close\"" w280 {
                  tunnel: w283 -> [w287 w300]
                  tunnel: [w289 w301] -> w282
                  tunnel: w281 -> [w288 w298]
                  frame "Open", Default {
                    n117 = property class="VI"(reference=w288, error in=w287) -> (reference out=w285:refnum<vi>, error out=w286:errorcluster, "FP.State"=w284:T3)
                    n118 = case shown="\"Closed\"" w284 {
                      tunnel: [w292 w295] -> w289
                      tunnel: w286 -> [w291 w295]
                      tunnel: w285 -> [w290 _]
                      frame "Closed" {
                        n119 = invoke class="VI" method="FP.Open"(reference=w290, error in=w291, "Activate"=TRUE, "State"=T3."Standard") -> (error out=w292:errorcluster)  [unwired: 1 in, 4 out]
                      }
                      frame Default {
                      }
                    }
                  }
                  frame "Close" {
                    n120 = property class="VI"(reference=w298, error in=w300) -> (reference out=w297:refnum<vi>, error out=w299:errorcluster, "FP.State"=w296:T3)
                    n121 = case shown="Default" w296 {
                      tunnel: [w302 w305] -> w301
                      tunnel: w299 -> [w302 w304]
                      tunnel: w297 -> [_ w303]
                      frame "Invalid", "Closed" {
                      }
                      frame Default {
                        n122 = invoke class="VI" method="FP.Close"(reference=w303, error in=w304) -> (error out=w305:errorcluster)  [unwired: 1 in, 2 out]
                      }
                    }
                  }
                }
              }
              frame condition #1 {
              }
            }
            n123 = call <vilib>:"Add State(s) to Queue__jki_lib_state_machine.vi"("State(s) in (\"\")"=w279) -> ("States Out"=w278:string)  [unwired: 14 in]
          }
          frame "UI: Update Graphs" {
            n124 = Unbundle By Name(w315) -> ("SMU Data"=w314:cluster{"X":dbl, "Y":dbl}[], "LIA Data"=w313:cluster{"X":dbl, "Y":dbl}[], "OPM Data"=w312:cluster{"X":dbl, "Y":dbl}[])
            n125 = property on="SMU" class="XYGraph (strict)"(error in=w311, "Value"=w314) -> (error out=w310:errorcluster)  [unwired: 1 in, 1 out]
            n126 = property on="LIA" class="XYGraph (strict)"(error in=w311, "Value"=w313) -> (error out=w309:errorcluster)  [unwired: 1 in, 1 out]
            n127 = property on="Power monitor" class="XYGraph (strict)"(error in=w311, "Value"=w312) -> (error out=w308:errorcluster)  [unwired: 1 in, 1 out]
            n128 = Merge Errors(w310, w309, w308) -> (w307:errorcluster)
            n129 = call <vilib>:"Add State(s) to Queue__jki_lib_state_machine.vi"("State(s) in (\"\")"=w318) -> ("States Out"=w317:string)  [unwired: 14 in]
          }
          frame "---------- Macro ----------" {
            # "Do not put any code in this frame.\n(It is a separator no-op. You can make a copy of this frame to create a new Macro frame)"
            n130 = call <vilib>:"Add State(s) to Queue__jki_lib_state_machine.vi"("State(s) in (\"\")"=w323) -> ("States Out"=w322:string)  [unwired: 14 in]
          }
          frame "Macro: Initialize" {
            w326 = "UI: Initialize\n//UI: Front Panel State >> Open"  # UI: Initialize //UI: Front Panel State >> Open
            # "Initialization Macro\n(This is called once, when the VI starts)"
            n131 = call <vilib>:"Add State(s) to Queue__jki_lib_state_machine.vi"("State(s) in Front (\"\")"="Data: Initialize\nInitialize Core Data\nEvents: Register", "State(s) in (\"\")"="Process: Sync", "State(s) at Back (\"\")"=w326) -> ("States Out"=w325:string)  [unwired: 12 in]
            n132 = call <vilib>:"Add State(s) to Queue__jki_lib_state_machine.vi"("State(s) in Front (\"\")"=w325, "State(s) in (\"\")"=w332) -> ("States Out"=w331:string)  [unwired: 13 in]
          }
          frame "Macro: Exit" {
            # "Exit Macro\n(This is called once, when the VI exits)"
            n133 = Unbundle By Name(w337) -> ("Core.Close Panel on Exit?"=w343:bool)
            n134 = Select(t="//UI: Front Panel State >> Close", s=w343, f="") -> (s? t:f=w340:string)
            n135 = call <vilib>:"Add State(s) to Queue__jki_lib_state_machine.vi"("State(s) in Front (\"\")"="Data: Cleanup\nEvents: Unregister", "State(s) in (\"\")"="Process: Sync", "State(s) at Back (\"\")"="Exit") -> ("States Out"=w334:string)  [unwired: 12 in]
            n136 = call <vilib>:"Add State(s) to Queue__jki_lib_state_machine.vi"("State(s) in (\"\")"=w340, "State(s) at Back (\"\")"=w334) -> ("States Out"=w339:string)  [unwired: 13 in]
            n137 = call <vilib>:"Add State(s) to Queue__jki_lib_state_machine.vi"("State(s) in Front (\"\")"=w339, "State(s) in (\"\")"=w346) -> ("States Out"=w345:string)  [unwired: 13 in]
          }
          frame "---------- Process ----------" {
            # "Template Separator\n(You can make a copy of, or modify, this frame)"
            n138 = call <vilib>:"Add State(s) to Queue__jki_lib_state_machine.vi"("State(s) in (\"\")"=w351) -> ("States Out"=w350:string)  [unwired: 14 in]
          }
          frame "Process: Sync" {
            n139 = Unbundle By Name(w359) -> ("Self Reference"=w355:refnum<class "Measurement.Free.UI.lvclass">)
            n140 = call <vilib>:"WaitOnProcessSync.vi"("error in (no error)"=w354, "SMO"=w355) -> ("error out"=w353:errorcluster, "Don't run?"=w358:bool)  [unwired: 7 in, 1 out]
            n141 = Select(t="Data: Cleanup\nEvents: Unregister\nExit", s=w358, f="") -> (s? t:f=w352:string)
            n142 = call <vilib>:"Add State(s) to Queue__jki_lib_state_machine.vi"("State(s) in Front (\"\")"=w352, "State(s) in (\"\")"=w362) -> ("States Out"=w361:string)  [unwired: 13 in]
          }
          frame "---------- Events ----------" {
            # "Template Separator\n(You can make a copy of, or modify, this frame)"
            n143 = call <vilib>:"Add State(s) to Queue__jki_lib_state_machine.vi"("State(s) in (\"\")"=w367) -> ("States Out"=w366:string)  [unwired: 14 in]
          }
          frame "Events: Register" {
            # "Measurement base class Public Events"
            # "Base Class Protected Events"
            n144 = Unbundle By Name(w373) -> ("Self Reference"=w374:refnum<class "Measurement.Free.UI.lvclass">)
            n145 = Unbundle By Name(w373) -> ("Dependencies.Measurement.Free"=w370:refnum<class "Measurement.Free.lvclass">)
            n146 = call <vilib>:"GetProtectedEvents.vi"("SMO"=w374) -> ("error out"=w375:errorcluster, "SMO Protected Events"=w379:T9)  [unwired: 8 in, 1 out]
            n147 = call "Measurement.GetPublicEventsRegistration.vi"("Measurement in"=w370) -> ("error out"=w368:errorcluster, "Measurement Public Events"=w369:refnum<event-registration>)  [unwired: 8 in, 1 out]
            n148 = register-events(w379) -> (reference out=w372:refnum<event-registration>, error out=w377:errorcluster)  [unwired: 2 in]
            n149 = Bundle("Event Registration Refnum"=w372, "Measurement Public Events"=w369) -> (w371:T10)  [unwired: 1 in]
            n150 = Merge Errors(w378, w377, w375, w368) -> (w376:errorcluster)
            n151 = call <vilib>:"Add State(s) to Queue__jki_lib_state_machine.vi"("State(s) in (\"\")"=w381) -> ("States Out"=w380:string)  [unwired: 14 in]
          }
          frame "Events: Unregister" {
            n152 = Unregister For Events(event registration refnum=w384, error in=w383) -> (error out=w382:errorcluster)
            n153 = call <vilib>:"Add State(s) to Queue__jki_lib_state_machine.vi"("State(s) in (\"\")"=w387) -> ("States Out"=w386:string)  [unwired: 14 in]
          }
          frame "---------- Action ----------" {
            n154 = Unbundle By Name(w390) -> ("Self Reference"=w388:refnum<class "Measurement.Free.UI.lvclass">)
            n155 = Bundle By Name(cluster=w390, "Self Reference"=w388) -> (w389:T7)
            n156 = call <vilib>:"Add State(s) to Queue__jki_lib_state_machine.vi"("State(s) in (\"\")"=w394) -> ("States Out"=w393:string)  [unwired: 14 in]
          }
          frame "Action: Notify UI Closed" {
            # "Notify that the UI has been closed"
            n157 = Unbundle By Name(w397) -> ("Self Reference"=w398:refnum<class "Measurement.Free.UI.lvclass">)
            n158 = call <vilib>:"Hide.vi"("error in (no error)"=w396, "SMO.UI"=w398) -> ("error out"=w395:errorcluster)  [unwired: 8 in, 1 out]
            n159 = call <vilib>:"Add State(s) to Queue__jki_lib_state_machine.vi"("State(s) in (\"\")"=w401) -> ("States Out"=w400:string)  [unwired: 14 in]
          }
        }
      }
    }
    frame Error {
    }
  }
  n160 = call-parent "Process.vi"("error in (no error)"=w8, "SMO.UI"=w7) -> ("error out"=w5:errorcluster, "SMO.UI out"=→"Measurement.Free.UI out":refnum<class "Measurement.Free.UI.lvclass">)  [unwired: 8 in]
  n161 = Merge Errors(w5, w4) -> (→"error out":errorcluster)
